vi "calculatoLV2021.vi"() -> ()   [LabVIEW 2021]
panel:
  out "Wyjscie":string
  in  "Clear":bool
  in  "Enter":bool
  in  "Divide":bool
  in  "Multiply":bool
  in  "Minus":bool
  in  "Plus":bool
  in  "X":dbl
  out "Z":dbl
  out "Y":dbl
  in  "Klawiatura numeryczna":T1
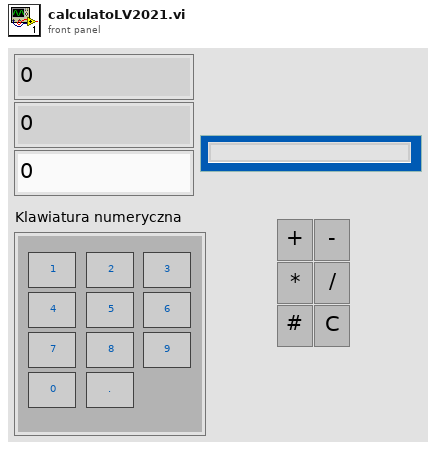
[diagram p1: front panel]
types:
  T1 = cluster{"1":bool, "2":bool, "3":bool, "4":bool, "5":bool, "6":bool, "7":bool, "8":bool, "9":bool, "0":bool, ".":bool}
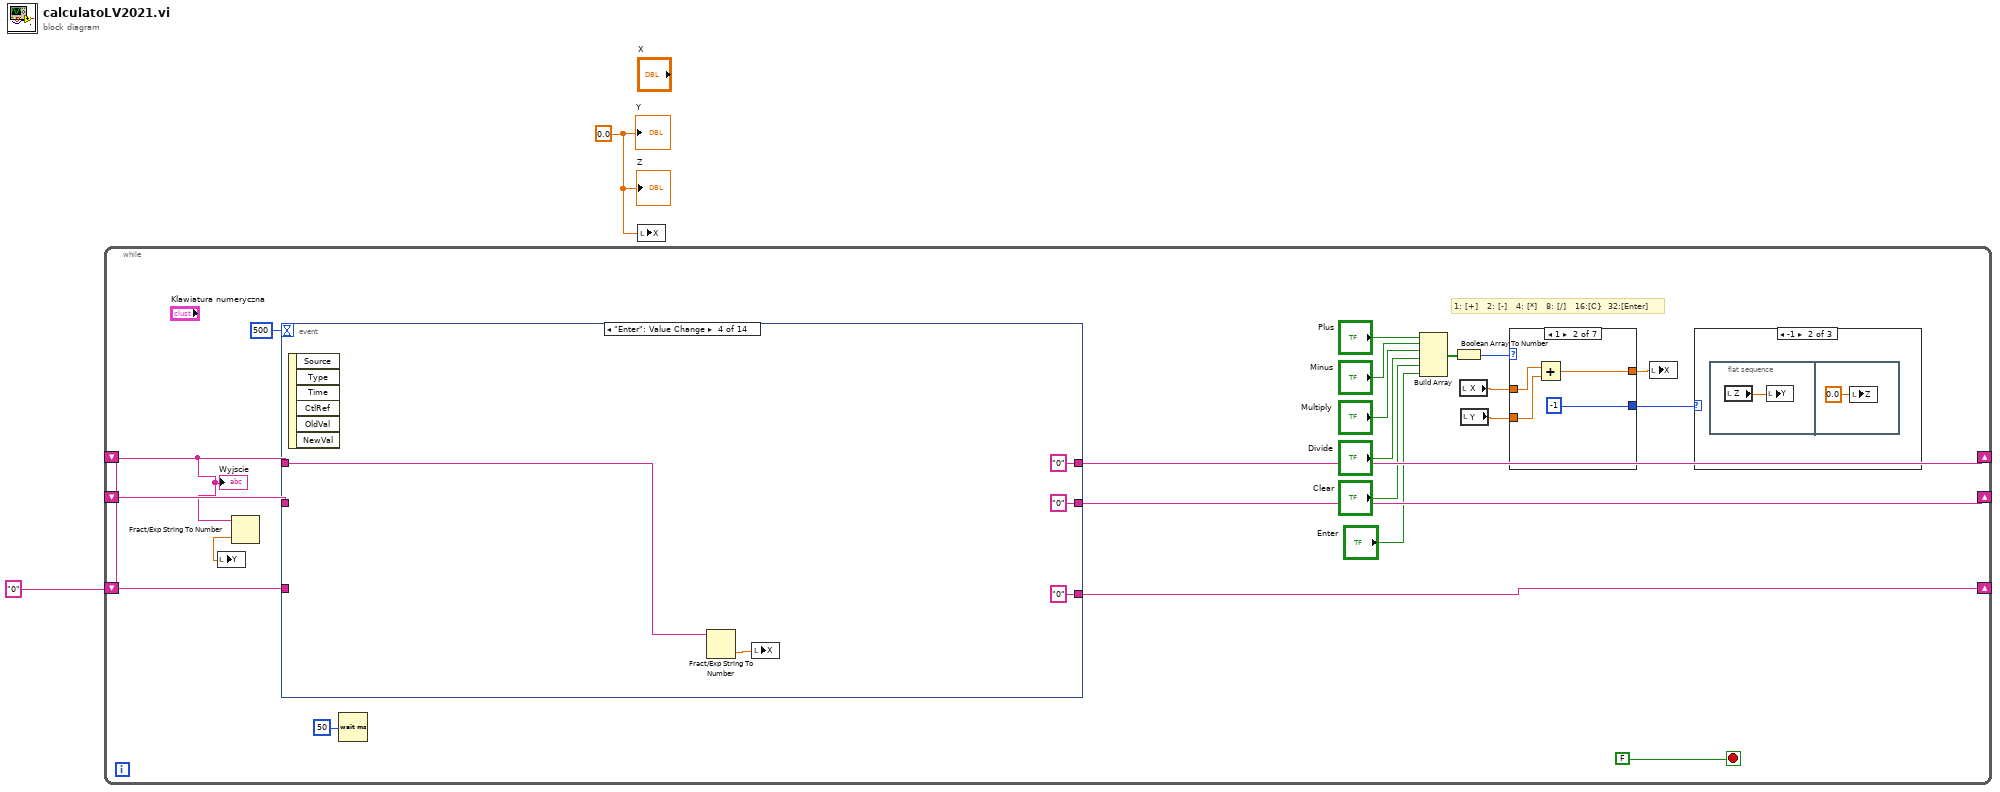
[diagram p0: block diagram]
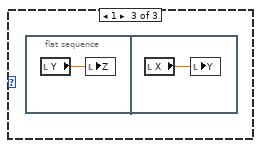
[diagram p3: hidden frame]
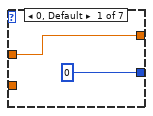
[diagram p4: hidden frame]
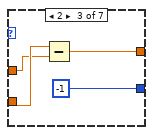
[diagram p5: hidden frame]
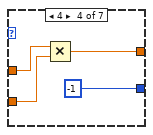
[diagram p6: hidden frame]
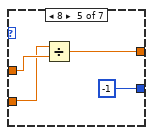
[diagram p7: hidden frame]
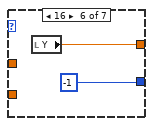
[diagram p8: hidden frame]
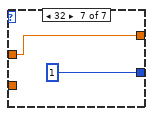
[diagram p9: hidden frame]
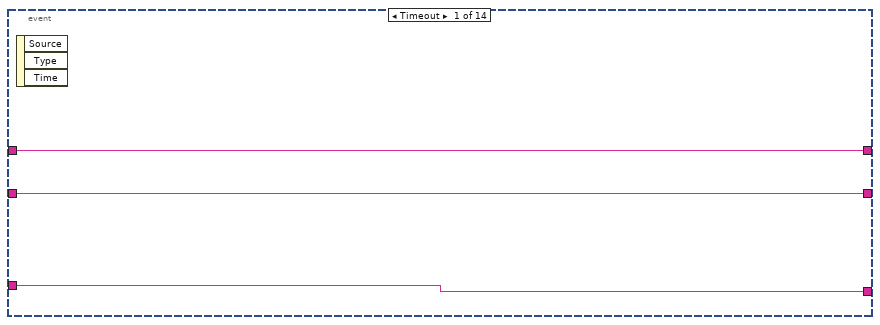
[diagram p10: hidden frame]
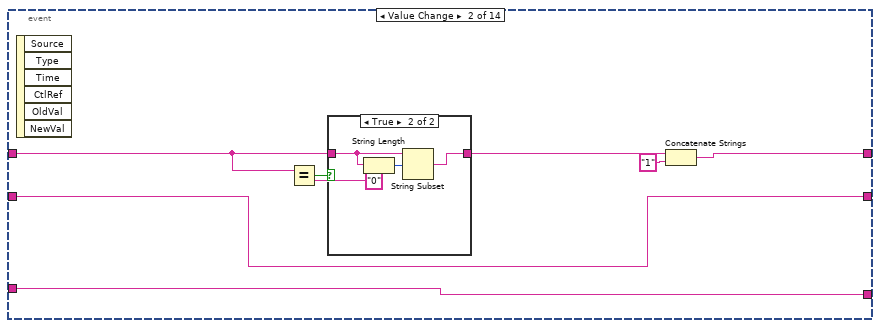
[diagram p11: hidden frame]
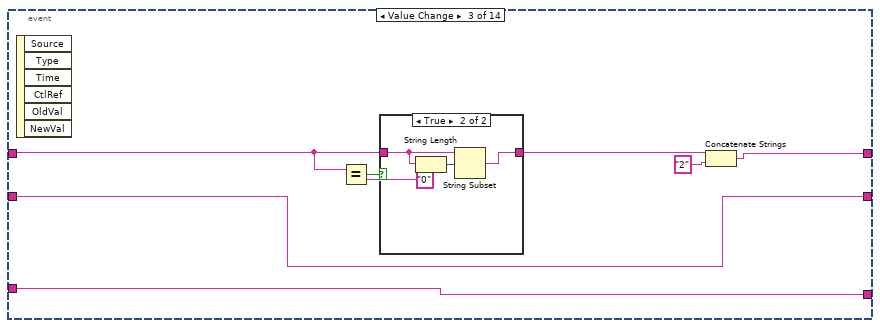
[diagram p13: hidden frame]
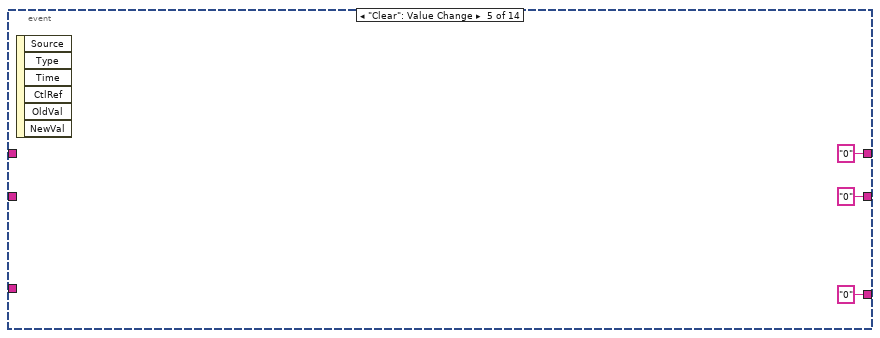
[diagram p15: hidden frame]
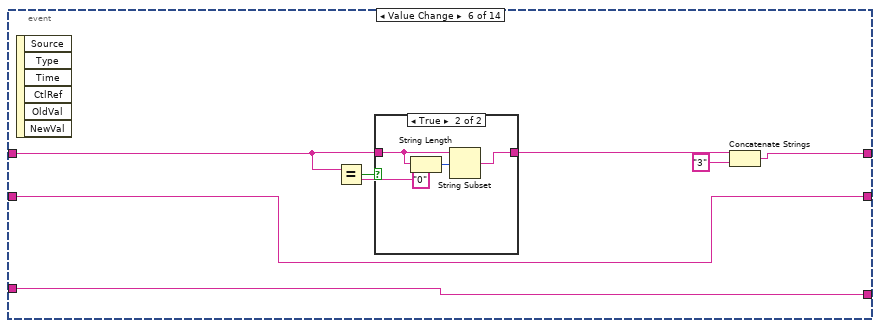
[diagram p16: hidden frame]
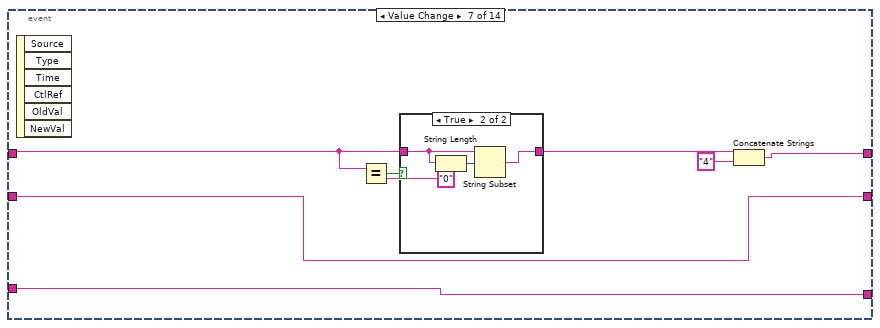
[diagram p18: hidden frame]
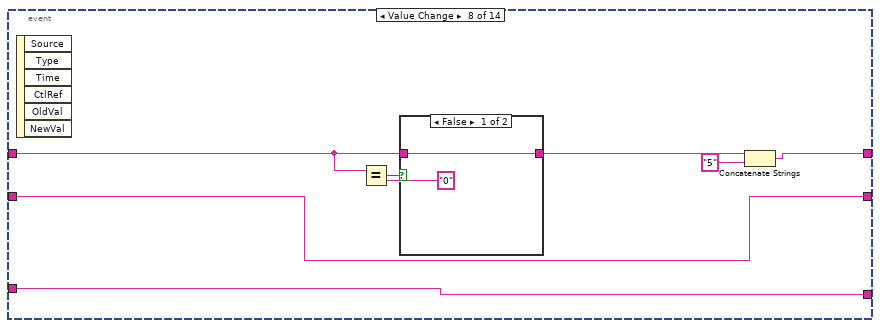
[diagram p20: hidden frame]
diagram:
  w1 = 0.0 ("Y")
  w2 = "0"
  n1 = while {
    shift-right: [w17] -> _
    shift-left: w2 -> [w4]
    shift-right: [w18] -> _
    shift-left: w2 -> [w20]
    shift-right: [w19] -> _
    shift-left: w2 -> [w21]
    stop <- FALSE ("Enter 2") stop-if-true
    # "1: [+]   2: [-]   4: [*]   8: [/]   16:[C}  32:[Enter]"
    n2 = Fract/Exp String To Number(string=w4) -> (number=w3:dbl)  [unwired: 3 in, 1 out]
    n3 = local write "Y"(w3) -> ()
    n4 = event shown="[3] \"Enter\": Value Change" {
      selector: _ -> [_ _ _ _ _ _ _ _ _ _ _ _ _ _]
      dyn-events: _ -> [_ _ _ _ _ _ _ _ _ _ _ _ _ _]
      timeout: 500 -> [_ _ _ _ _ _ _ _ _ _ _ _ _ _]
      tunnel: w4 -> [w52 w55 w67 w81 _ w87 w100 w111 w123 w135 w147 w159 w174 w178]
      tunnel: [w53 w60 w72 "0" "0" w92 w104 w116 w129 w140 w152 w164 w172 w179] -> w18
      tunnel: w20 -> [w53 w60 w72 _ _ w92 w104 w116 w129 w140 w152 w164 w172 w179]
      tunnel: [w52 w59 w71 "0" "0" w91 w103 w115 w128 w139 w151 w163 w171 w177] -> w17
      tunnel: [w51 w54 w66 "0" "0" w86 w98 w110 w122 w134 w146 w158 w170 w175] -> w19
      tunnel: w21 -> [w51 w54 w66 _ _ w86 w98 w110 w122 w134 w146 w158 w170 w175]
      event Timeout {
        n5 = event-data() -> ()  [unwired: 1 in, 3 out]
      }
      event "Klawiatura numeryczna.1": Value Change {
        n6 = event-data() -> ()  [unwired: 1 in, 6 out]
        n7 = Equal?(x=w55, y="0") -> (x = y?=w58:bool)
        n8 = case shown="True" w58 {
          tunnel: w55 -> [w62 w64]
          tunnel: [w62 w63] -> w56
          frame False {
          }
          frame True {
            n9 = String Length(string=w64) -> (length=w65:i32)
            n10 = String Subset(string=w64, offset (0)=w65) -> (substring=w63:string)  [unwired: 1 in]
          }
        }
        n11 = Concatenate Strings(w56, "1") -> (w59:string)
      }
      event "Klawiatura numeryczna.2": Value Change {
        n12 = event-data() -> ()  [unwired: 1 in, 6 out]
        n13 = Equal?(x=w67, y="0") -> (x = y?=w70:bool)
        n14 = case shown="True" w70 {
          tunnel: w67 -> [w74 w76]
          tunnel: [w74 w75] -> w68
          frame False {
          }
          frame True {
            n15 = String Length(string=w76) -> (length=w77:i32)
            n16 = String Subset(string=w76, offset (0)=w77) -> (substring=w75:string)  [unwired: 1 in]
          }
        }
        n17 = Concatenate Strings(w68, "2") -> (w71:string)
      }
      event "Enter": Value Change {
        n18 = event-data() -> ()  [unwired: 1 in, 6 out]
        n19 = Fract/Exp String To Number(string=w81) -> (number=w82:dbl)  [unwired: 3 in, 1 out]
        n20 = local write "X"(w82) -> ()
      }
      event "Clear": Value Change {
        n21 = event-data() -> ()  [unwired: 1 in, 6 out]
      }
      event "Klawiatura numeryczna.3": Value Change {
        n22 = event-data() -> ()  [unwired: 1 in, 6 out]
        n23 = Equal?(x=w87, y="0") -> (x = y?=w90:bool)
        n24 = case shown="True" w90 {
          tunnel: w87 -> [w94 w96]
          tunnel: [w94 w95] -> w88
          frame False {
          }
          frame True {
            n25 = String Length(string=w96) -> (length=w97:i32)
            n26 = String Subset(string=w96, offset (0)=w97) -> (substring=w95:string)  [unwired: 1 in]
          }
        }
        n27 = Concatenate Strings(w88, "3") -> (w91:string)
      }
      event "Klawiatura numeryczna.4": Value Change {
        n28 = event-data() -> ()  [unwired: 1 in, 6 out]
        n29 = Equal?(x=w100, y="0") -> (x = y?=w102:bool)
        n30 = case shown="True" w102 {
          tunnel: w100 -> [w106 w108]
          tunnel: [w106 w107] -> w99
          frame False {
          }
          frame True {
            n31 = String Length(string=w108) -> (length=w109:i32)
            n32 = String Subset(string=w108, offset (0)=w109) -> (substring=w107:string)  [unwired: 1 in]
          }
        }
        n33 = Concatenate Strings(w99, "4") -> (w103:string)
      }
      event "Klawiatura numeryczna.5": Value Change {
        n34 = event-data() -> ()  [unwired: 1 in, 6 out]
        n35 = Equal?(x=w111, y="0") -> (x = y?=w114:bool)
        n36 = case shown="False" w114 {
          tunnel: w111 -> [w118 w120]
          tunnel: [w118 w119] -> w112
          frame False {
          }
          frame True {
            n37 = String Length(string=w120) -> (length=w121:i32)
            n38 = String Subset(string=w120, offset (0)=w121) -> (substring=w119:string)  [unwired: 1 in]
          }
        }
        n39 = Concatenate Strings(w112, "5") -> (w115:string)
      }
      event "Klawiatura numeryczna.6": Value Change {
        n40 = event-data() -> ()  [unwired: 1 in, 6 out]
        n41 = Equal?(x=w123, y="0") -> (x = y?=w126:bool)
        n42 = case shown="True" w126 {
          tunnel: w123 -> [w130 w132]
          tunnel: [w130 w131] -> w124
          frame False {
          }
          frame True {
            n43 = String Length(string=w132) -> (length=w133:i32)
            n44 = String Subset(string=w132, offset (0)=w133) -> (substring=w131:string)  [unwired: 1 in]
          }
        }
        n45 = Concatenate Strings(w124, "6") -> (w128:string)
      }
      event "Klawiatura numeryczna.7": Value Change {
        n46 = event-data() -> ()  [unwired: 1 in, 6 out]
        n47 = Equal?(x=w135, y="0") -> (x = y?=w138:bool)
        n48 = case shown="True" w138 {
          tunnel: w135 -> [w142 w144]
          tunnel: [w142 w143] -> w136
          frame False {
          }
          frame True {
            n49 = String Length(string=w144) -> (length=w145:i32)
            n50 = String Subset(string=w144, offset (0)=w145) -> (substring=w143:string)  [unwired: 1 in]
          }
        }
        n51 = Concatenate Strings(w136, "7") -> (w139:string)
      }
      event "Klawiatura numeryczna.8": Value Change {
        n52 = event-data() -> ()  [unwired: 1 in, 6 out]
        n53 = Equal?(x=w147, y="0") -> (x = y?=w150:bool)
        n54 = case shown="True" w150 {
          tunnel: w147 -> [w154 w156]
          tunnel: [w154 w155] -> w148
          frame False {
          }
          frame True {
            n55 = String Length(string=w156) -> (length=w157:i32)
            n56 = String Subset(string=w156, offset (0)=w157) -> (substring=w155:string)  [unwired: 1 in]
          }
        }
        n57 = Concatenate Strings(w148, "8") -> (w151:string)
      }
      event "Klawiatura numeryczna.9": Value Change {
        n58 = event-data() -> ()  [unwired: 1 in, 6 out]
        n59 = Equal?(x=w159, y="0") -> (x = y?=w162:bool)
        n60 = case shown="True" w162 {
          tunnel: w159 -> [w166 w168]
          tunnel: [w166 w167] -> w160
          frame False {
          }
          frame True {
            n61 = String Length(string=w168) -> (length=w169:i32)
            n62 = String Subset(string=w168, offset (0)=w169) -> (substring=w167:string)  [unwired: 1 in]
          }
        }
        n63 = Concatenate Strings(w160, "9") -> (w163:string)
      }
      event "Klawiatura numeryczna.0": Value Change {
        n64 = event-data() -> ()  [unwired: 1 in, 6 out]
        n65 = Concatenate Strings(w174, "0") -> (w171:string)
      }
      event "Klawiatura numeryczna..": Value Change {
        n66 = event-data() -> ()  [unwired: 1 in, 6 out]
        n67 = Concatenate Strings(w178, "." ("string")) -> (w177:string)
      }
    }
    n68 = Wait (ms)(milliseconds to wait=u32 50) -> ()  [unwired: 1 out]
    n69 = Build Array("Plus", "Minus", "Multiply", "Divide", "Clear", "Enter") -> (w12:bool[])
    n70 = Boolean Array To Number(Boolean array=w12) -> (number=w7:u32)
    n71 = local read "X"() -> (w10:dbl)
    n72 = local read "Y"() -> (w8:dbl)
    n73 = case shown="1" w7 {
      tunnel: w8 -> [_ w34 w37 w41 w44 _ _]
      tunnel: [w30 w33 w38 w40 w46 w47 w49] -> w9
      tunnel: w10 -> [w30 w32 w36 w42 w45 _ w49]
      tunnel: [0 -1 -1 -1 -1 -1 1] -> w5
      frame 0, Default {
      }
      frame 1 {
        n74 = Add(x=w32, y=w34) -> (x+y=w33:dbl)
      }
      frame 2 {
        n75 = Subtract(x=w37, y=w36) -> (x-y=w38:dbl)
      }
      frame 4 {
        n76 = Multiply(x=w42, y=w41) -> (x*y=w40:dbl)
      }
      frame 8 {
        n77 = Divide(x=w44, y=w45) -> (x/y=w46:dbl)
      }
      frame 16 {
        n78 = local read "Y"() -> (w47:dbl)
      }
      frame 32 {
      }
    }
    n79 = local write "X"(w9) -> ()
    n80 = case shown="-1" w5 {
      frame 0, Default {
      }
      frame -1 {
        n81 = flat-sequence {
          frame #0 {
            n82 = local read "Z"() -> (w25:dbl)
            n83 = local write "Y"(w25) -> ()
          }
          frame #1 {
            n84 = local write "Z"(0.0 ("Y")) -> ()
          }
        }
      }
      frame 1 {
        n85 = flat-sequence {
          frame #0 {
            n86 = local read "Y"() -> (w27:dbl)
            n87 = local write "Z"(w27) -> ()
          }
          frame #1 {
            n88 = local read "X"() -> (w28:dbl)
            n89 = local write "Y"(w28) -> ()
          }
        }
      }
    }
    "Wyjscie" <- w4
  }
  n90 = local write "X"(w1) -> ()
  "Y" <- w1
  "Z" <- w1
